vi "Get PID and Name.vi"(8 "error in (no error)":errorcluster) -> (0 "error out":errorcluster, 1 "Name":string, 2 "PID":u32)   [LabVIEW 2021, in "CIF Engine Launch.lvlib"]
uses:
  CIFLauncher/CIFLauncher.lvclass/CIFLauncher.ctl
  CIF Engine Launch.lvlib
  kernel32.dll
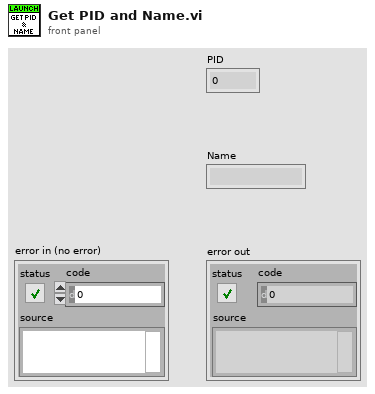
[diagram p1: front panel]
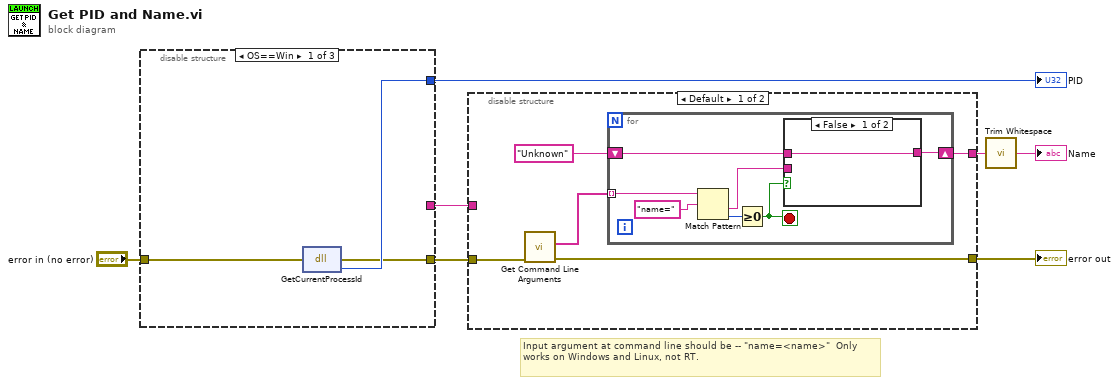
[diagram p0: block diagram]
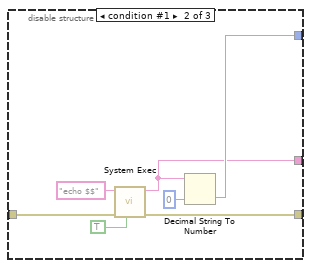
[diagram p2: hidden frame]
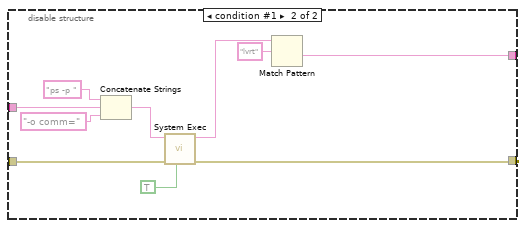
[diagram p5: hidden frame]
diagram:
  # "Input argument at command line should be -- \"name=<name>\"  Only works on Windows and Linux, not RT."
  n1 = disable-structure shown="OS==Win" {
    disable-tunnel: [w10 w14 _] -> w3
    disable-tunnel: [w9 w17 w18] -> w7
    disable-tunnel: [_ w12 _] -> w6
    disable-tunnel: "error in (no error)" -> [w8 w11 w18]
    frame condition #0 (active) {
      n2 = dll-call lib="kernel32.dll" fn="GetCurrentProcessId"(error in=w8) -> (error out=w9:errorcluster, "return type"=w10:u32)  [unwired: 2 in, 1 out]
    }
    frame condition #1 {
      n3 = call <vilib>:"System Exec.vi"("run minimized? (F)"=TRUE, "error in (no error)"=w11, "command line"="echo $$") -> ("error out"=w17:errorcluster, "standard output"=w12:string)  [unwired: 5 in, 2 out]
      n4 = Decimal String To Number(string=w12, default (0L)=u32 0 ("default (0 I32)")) -> (number=w14:u32)  [unwired: 1 in, 1 out]
    }
    frame condition #2 {
    }
  }
  "PID" <- w3
  n5 = disable-structure shown="Default" {
    disable-tunnel: [w21 w33] -> w2
    disable-tunnel: w7 -> [w20 w41]
    disable-tunnel: w6 -> [_ w39]
    disable-tunnel: [w19 w36] -> w4
    frame condition #0 (active) {
      n6 = call <vilib>:"Get Command Line Arguments.vi"("error in (no error)"=w20) -> ("error out"=w19:errorcluster, "arguments"=w23:string[])  [unwired: 8 in, 1 out]
      n7 = for {
        tunnel: w23 -> [w30] mode=indexing
        shift-right: [w24] -> w21
        shift-left: "Unknown" -> [w27]
        stop <- w26 stop-if-true
        n8 = Match Pattern(string=w30, regular expression="name=") -> (after substring=w25:string, offset past match=w28:i32)  [unwired: 1 in, 2 out]
        n9 = Greater Or Equal To 0?(x=w28) -> (x >= 0?=w26:bool)
        n10 = case shown="False" w26 {
          tunnel: w27 -> [w31 _]
          tunnel: w25 -> [_ w32]
          tunnel: [w31 w32] -> w24
          frame False {
          }
          frame True {
          }
        }
      }
    }
    frame condition #1 {
      n11 = Concatenate Strings("ps -p " ("string"), w39, "-o comm=" ("string")) -> (w37:string)
      n12 = call <vilib>:"System Exec.vi"("run minimized? (F)"=TRUE, "error in (no error)"=w41, "command line"=w37) -> ("error out"=w36:errorcluster, "standard output"=w35:string)  [unwired: 5 in, 2 out]
      n13 = Match Pattern(string=w35, regular expression="lvrt") -> (after substring=w33:string)  [unwired: 1 in, 3 out]
    }
  }
  "error out" <- w4
  n14 = call <vilib>:"Trim Whitespace.vi"("string"=w2) -> ("trimmed string"=→"Name":string)  [unwired: 1 in]
